vi "Robot_Targeting_adjustment.vi"   [LabVIEW 2017]
panel:
  # ".7\n-.7"
  # "1\n-1"
  # ".5\n-.5"
  # "Rotation"
  # "Strafe"
  # "Forward back"
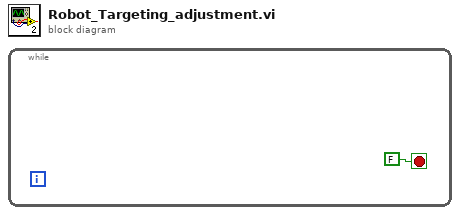
[diagram p0: block diagram]
diagram:
  n1 = while {
    stop <- FALSE stop-if-true
  }
